vi "Averaged DC-RMS for 1 Chan.vi"(6 "averaging control":T2={"window for DC"=enum."Rectangular (none)", "output function"=enum."DC and RMS", "window for RMS"=enum."Rectangular (none)", "exp. time constant"=-1.0, "Ignore input start time"=FALSE} {"exp. time constant" format="%0.2p"}, 7 "reset":bool, 8 "error in (no error)":errorcluster, 9 "averaging time":dbl=-1.0 format="%0.2p", 10 "averaging type":enum16{"Linear", "Exponential"}(ring), 11 "signal in":waveform(dbl)) -> (0 "error out":errorcluster, 2 "RMS value waveform":waveform(dbl), 3 "DC value waveform":waveform(dbl), 4 "measurement info":T1={"uncertainty"=0.0, "Warning"=FALSE, "comments"="reserved for future use"} {"uncertainty" format="%0.2p"}, 5 "data ready":bool)   [LabVIEW 2020, in "NI_MAPro.lvlib"]
doc: "Calculates the DC and RMS values of an input waveform or array of waveforms. This VI is similar to the Basic Averaged DC-RMS VI, but this VI gives more precise control over the individual DC and RMS calculations."
uses:
  NI_MAPro.lvlib
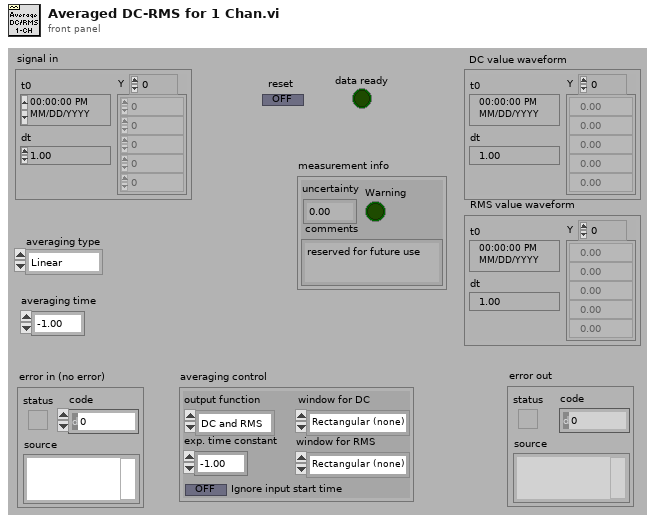
[diagram p1: front panel]
types:
  T1 = cluster{"uncertainty":dbl, "Warning":bool, "comments":string}
  T2 = cluster{"window for DC":enum16{"Rectangular (none)", "Hanning", "Low side lobe"}, "output function":enum16{"DC only", "RMS only", "DC and RMS"}, "window for RMS":enum16{"Rectangular (none)", "Hanning", "Low side lobe"}, "exp. time constant":dbl, "Ignore input start time":bool}
  T3 = cluster{"DC history":dbl, "RMS history":dbl, "exp TC (samples)":dbl, "buffer size":i32, "t0 history":timestamp, "dt history":dbl, "timestamp":timestamp, "buffer":dbl[]}
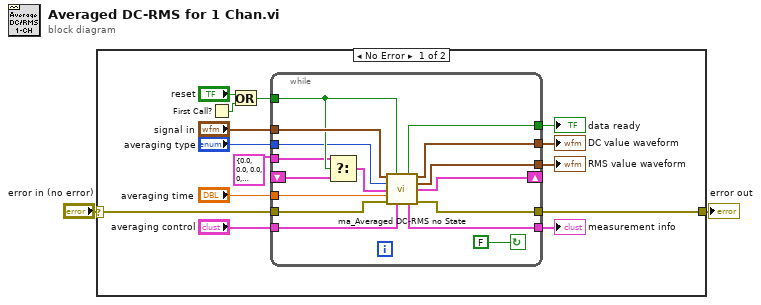
[diagram p0: block diagram]
diagram:
  n1 = case shown="No Error" "error in (no error)" {
    selector: "error in (no error)" -> [w3 w33]
    tunnel: [w16 w33] -> w2
    frame No Error {
      n2 = First Call?() -> (First Call?: T/F=w12:bool)
      n3 = Or(x="reset", y=w12) -> (x .or. y?=w11:bool)
      n4 = while {
        tunnel: [w19] -> w5
        tunnel: "averaging control" -> [w25]
        tunnel: T3 {"DC history"=0.0, "RMS history"=0.0, "exp TC (samples)"=0.0, "buffer size"=0, "t0 history"=timestamp(0 s since 1904-01-01), "dt history"=0.0, "timestamp"=timestamp(0 s since 1904-01-01), "buffer"=[]} ("state info") -> [w22]
        shift-left: _ -> [w21]
        shift-right: [w29] -> _
        tunnel: [w27] -> w16
        tunnel: w3 -> [w28]
        tunnel: "averaging type" -> [w18]
        tunnel: [w20] -> w7
        tunnel: "signal in" -> [w24]
        tunnel: "averaging time" -> [w30]
        tunnel: [w31] -> w15
        tunnel: [w32] -> w14
        tunnel: w11 -> [w23]
        stop <- FALSE continue-if-true
        n5 = Select(t=w22, s=w23, f=w21) -> (s? t:f=w17:T3)
        n6 = call "ma_Averaged DC-RMS no State.vi"("signal in"=w24, "reset"=w23, "averaging type"=w18, "state info"=w17, "averaging time"=w30, "error in"=w28, "averaging control"=w25) -> ("data ready"=w20:bool, "DC value waveform"=w31:waveform(dbl), "RMS value waveform"=w32:waveform(dbl), "state info"=w29:T3, "measurement info cluster"=w19:T1, "error out"=w27:errorcluster)  [unwired: 3 in]
      }
      "data ready" <- w7
      "DC value waveform" <- w15
      "RMS value waveform" <- w14
      "measurement info" <- w5
    }
    frame Error {
    }
  }
  "error out" <- w2
